vi "DetectorStart.vi"(8 "error in (no error)":errorcluster, 11 "Microscope in":refnum<class "Microscope.lvclass">) -> (0 "error out":errorcluster, 3 "Microscope out":refnum<class "Microscope.lvclass">)   [LabVIEW 2012, in "Microscope.lvclass"]
uses:
  classes/Microscope.lvclass
  classes/Microscope.lvclass/Microscope.ctl
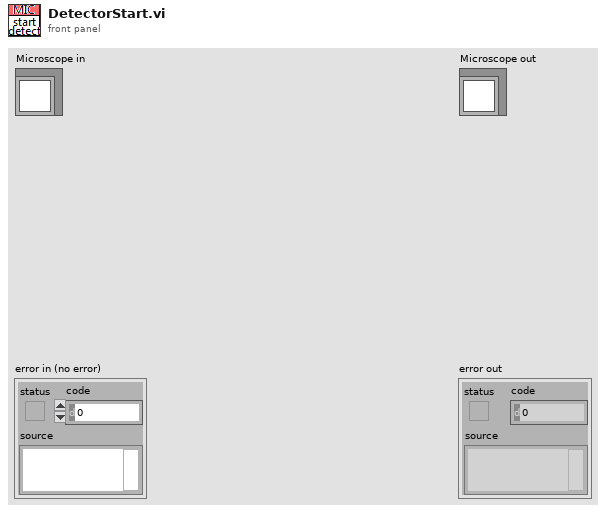
[diagram p1: front panel]
types:
  T1 = typedef "DetectorType.ctl" = enum16{"PMT", "SpectraWiz"}
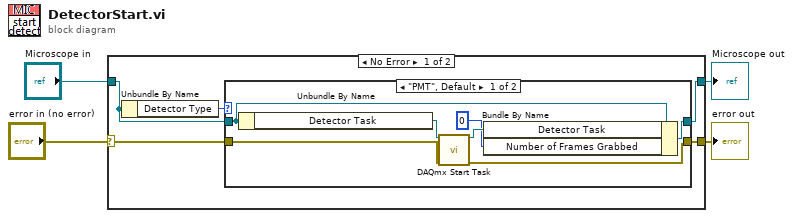
[diagram p0: block diagram]
diagram:
  n1 = case shown="No Error" "error in (no error)" {
    selector: "error in (no error)" -> [w7 w20]
    tunnel: [w8 w20] -> w3
    tunnel: [w9 w19] -> w1
    tunnel: "Microscope in" -> [w5 w19]
    frame No Error {
      n2 = Unbundle By Name(w5) -> ("Detector Type"=w6:T1)
      n3 = case shown="\"PMT\", Default" w6 {
        tunnel: [w14 w18] -> w9
        tunnel: [w13 w17] -> w8
        tunnel: w7 -> [w12 w17]
        tunnel: w5 -> [w10 w18]
        frame "PMT", Default {
          n4 = Unbundle By Name(w10) -> ("Detector Task"=w16:refnum<k21>)
          n5 = call <vilib>:"DAQmx Start Task.vi"("task/channels in"=w16, "error in"=w12) -> ("task out"=w15:refnum<k21>, "error out"=w13:errorcluster)  [unwired: 12 in]
          n6 = Bundle By Name(cluster=w10, "Detector Task"=w15, "Number of Frames Grabbed"=0) -> (w14:refnum<class "Microscope.lvclass">)
        }
        frame "SpectraWiz" {
        }
      }
    }
    frame Error {
    }
  }
  "error out" <- w3
  "Microscope out" <- w1
